vi "ReceiveAllPackets.vi"(8 "error in (no error)":errorcluster, 9 "ExpectedPacketCount":i32, 10 "EscapePattern":T1, 11 "VISA resource name":refnum<visa-resource-name>) -> (0 "error out":errorcluster, 2 "ReceivedBytes":T2[](array[typedef]), 3 "VISA resource name out":refnum<visa-resource-name>)   [LabVIEW 2009]
uses:
  Packet.ctl
  <vilib>/Instr/_visa.llb/VISA Flush IO Buffer Mask.ctl
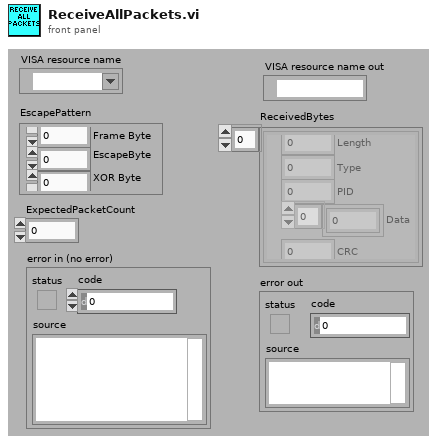
[diagram p1: front panel]
types:
  T1 = cluster{"Frame Byte":u8, "EscapeByte":u8, "XOR Byte":u8}
  T2 = typedef "Packet.ctl" = cluster{"Length":u8, "Type":u8, "PID":u8, "Data":u8[], "CRC":u8}
  T3 = typedef "VISA Flush IO Buffer Mask.ctl" = u16
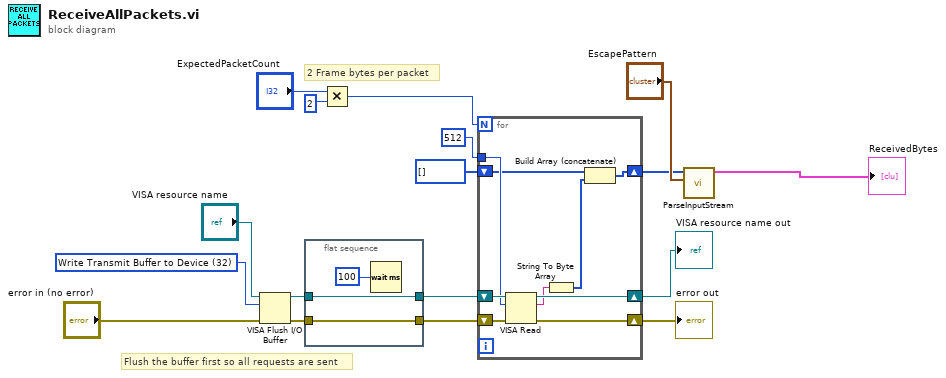
[diagram p0: block diagram]
diagram:
  w17 = T3 32 items=["Flush Receive Buffer"=16, "Write Transmit Buffer to Device"=32, "Flush Receive Buffer (No I/O)"=64, "Flush Transmit Buffer"=128] ("Mask")
  # "2 Frame bytes per packet"
  # "Flush the buffer first so all requests are sent"
  n1 = VISA Flush I/O Buffer(VISA resource name="VISA resource name", mask (16)=w17, error in (no error)="error in (no error)") -> (VISA resource name out=w12:refnum<visa-resource-name>, error out=w11:errorcluster)
  n2 = flat-sequence {
    tunnel: w12 -> [w20]
    tunnel: w11 -> [w19]
    tunnel: [w20] -> w10
    tunnel: [w19] -> w7
    frame #0 {
      n3 = Wait (ms)(milliseconds to wait=u32 100) -> ()  [unwired: 1 out]
    }
  }
  n4 = Multiply(x="ExpectedPacketCount", y=2) -> (x*y=w2:i32)
  n5 = for {
    N: w2 -> [_]
    tunnel: u32 512 ("byte count") -> [w28]
    shift-right: [w27] -> w8
    shift-left: w10 -> [w29]
    shift-right: [w21] -> w6
    shift-left: w7 -> [w25]
    shift-right: [w23] -> w4
    shift-left: u8[] [] ("unsigned byte array") -> [w24]
    n6 = VISA Read(VISA resource name=w29, byte count=w28, error in (no error)=w25) -> (VISA resource name out=w27:refnum<visa-resource-name>, read buffer=w26:string, error out=w21:errorcluster)  [unwired: 1 out]
    n7 = String To Byte Array(string=w26) -> (unsigned byte array=w22:u8[])
    n8 = Build Array (concatenate)(w24, w22) -> (w23:u8[])
  }
  "VISA resource name out" <- w8
  "error out" <- w6
  n9 = call "ParseInputStream.vi"("EscapePattern"="EscapePattern", "Data In"=w4) -> ("Array"=→"ReceivedBytes":T2[])  [unwired: 9 in]
